vi "2-2-3 Unflatten from JSON.vi"() -> ()   [LabVIEW 2020]
panel:
  out "JSON String Out":cluster{string, i32, dbl}
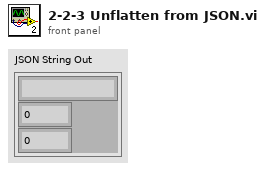
[diagram p1: front panel]
types:
  T1 = cluster{"status":string, "code":i32, "setpoint":dbl}
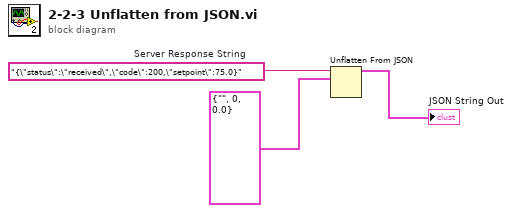
[diagram p0: block diagram]
diagram:
  w3 = "{\"status\":\"received\",\"code\":200,\"setpoint\":75.0}"  # Server Response String
  n1 = Unflatten From JSON(JSON string=w3, type and defaults=T1 {"status"="", "code"=0, "setpoint"=0.0}) -> (value=→"JSON String Out":T1)  [unwired: 5 in, 1 out]
